vi "Menu Selection.vi"(8 "error in (no error)":errorcluster, 10 "Tag":string, 11 "UserInterface in":refnum<class "UserInterface.lvclass">) -> (0 "error out":errorcluster, 3 "UserInterface out":refnum<class "UserInterface.lvclass">)   [LabVIEW 2016, in "UserInterface.lvlib" / "UserInterface.lvclass"]
doc: "Triggered when a right click menu item has been selected - determines which item has been selected and therefore what action needs to be taken - usually in the form of a message to be sent to the Assert Engine actor."
uses:
  UserInterface.lvclass
  C:/Program Files/National Instruments/LabVIEW 2016/vi.lib/ActorFramework/Actor/Actor.lvclass
  <vilib>/ActorFramework/Actor/Actor.lvclass/Actor.ctl
  AssertEngine/AssertEngine Messages/Update Assert Failure Action Msg/Update Assert Failure Action Msg.lvclass/Update Assert Failure Action Msg.ctl
  <vilib>/ActorFramework/Message Enqueuer/Message Enqueuer.lvclass/Message Enqueuer.ctl
  <vilib>/ActorFramework/Message Enqueuer/Enqueue.vi
  AssertEngine/AssertEngine Messages/Update Assert Failure Action Msg/Update Assert Failure Action Msg.lvclass
  C:/Program Files/National Instruments/LabVIEW 2016/vi.lib/ActorFramework/Message/Message.lvclass
  <vilib>/ActorFramework/Message Priority Queue/Priority Enqueue.vi
  <vilib>/ActorFramework/Actor/Actor.lvclass
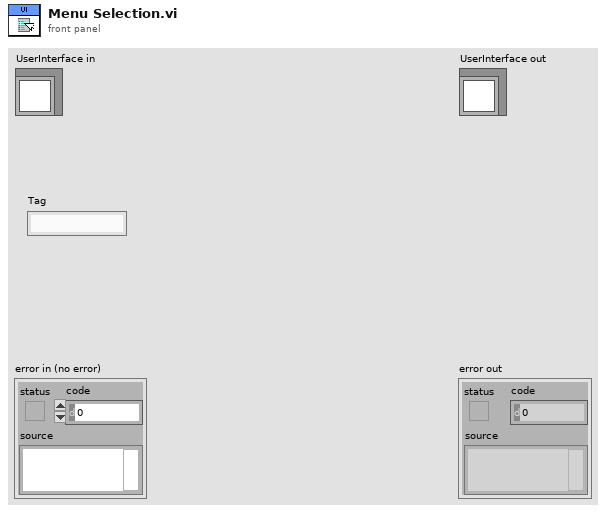
[diagram p1: front panel]
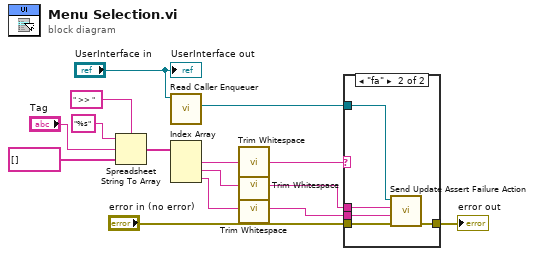
[diagram p0: block diagram]
diagram:
  n1 = Spreadsheet String To Array(delimiter (Tab)=" >> ", format string="%s", spreadsheet string="Tag", array type (2D Dbl)=string[] []) -> (array=w11:string[])
  n2 = call <vilib>:"Read Caller Enqueuer.vi"("Actor"="UserInterface in") -> ("Caller Enqueuer"=w9:refnum<class "Message Enqueuer.lvclass">)  [unwired: 10 in]
  n3 = Index Array(array=w11) -> (element #1=w4:string, element #2=w8:string, element #3=w7:string)  [unwired: 3 in]
  n4 = call <vilib>:"Trim Whitespace.vi"("string"=w4) -> ("trimmed string"=w3:string)  [unwired: 1 in]
  n5 = call <vilib>:"Trim Whitespace.vi"("string"=w8) -> ("trimmed string"=w2:string)  [unwired: 1 in]
  n6 = call <vilib>:"Trim Whitespace.vi"("string"=w7) -> ("trimmed string"=w1:string)  [unwired: 1 in]
  n7 = case shown="\"fa\"" w3 {
    tunnel: w9 -> [_ w21]
    tunnel: w2 -> [_ w20]
    tunnel: w1 -> [_ w19]
    tunnel: "error in (no error)" -> [w16 w18]
    tunnel: [w16 w17] -> w5
    frame Default {
    }
    frame "fa" {
      n8 = call "Send Update Assert Failure Action.vi"("error in (no error)"=w18, "Assert Name"=w19, "Target Failure Action"=w20, "Message Enqueuer"=w21) -> ("error out"=w17:errorcluster)  [unwired: 6 in, 1 out]
    }
  }
  "error out" <- w5
  "UserInterface out" <- "UserInterface in"
